vi "pp_sessList_save.vi"(8 "error in (no error)":errorcluster, 11 "Session List (Cannot Edit)":i32[](array[numeric])) -> (0 "error out":errorcluster, 3 "Session List File Path":path)   [LabVIEW 2013]
uses:
  <vilib>/Utility/file.llb/Write To Spreadsheet File (I64).vi
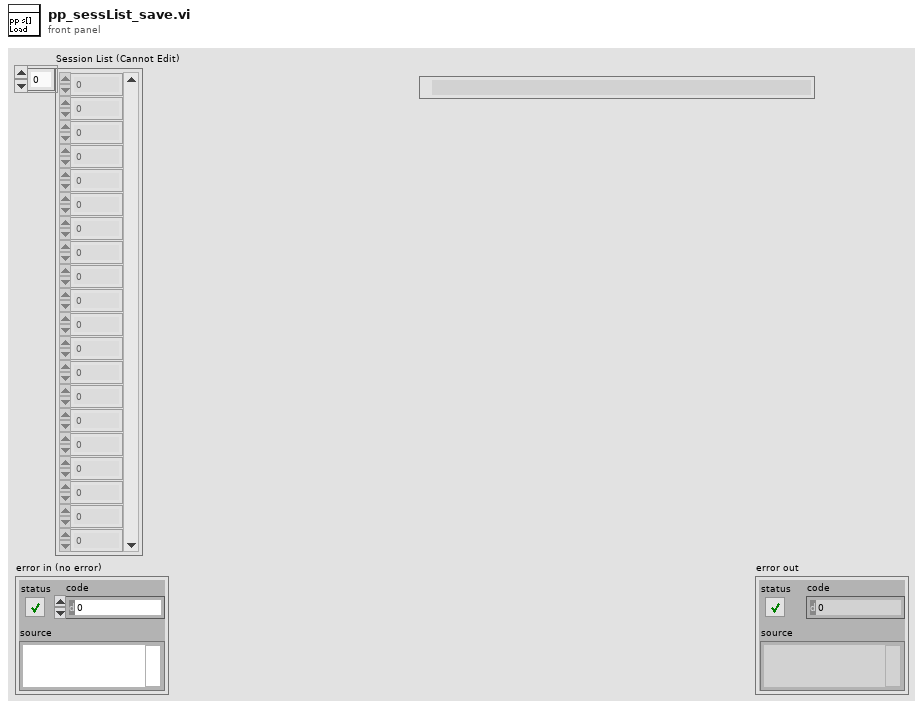
[diagram p1: front panel]
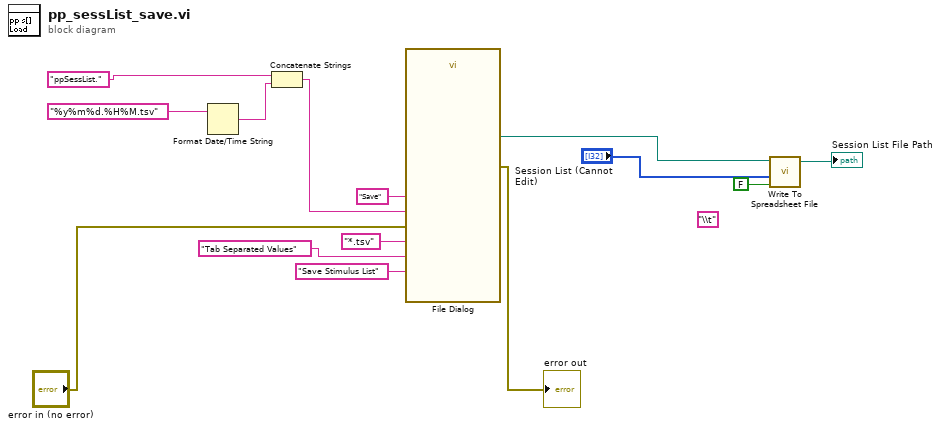
[diagram p0: block diagram]
diagram:
  (unwired) "\\t" ("delimiter (\\t)")
  n1 = Format Date/Time String(time format string (%c)="%y%m%d.%H%M.tsv") -> (date/time string=w10:string)  [unwired: 2 in]
  n2 = Concatenate Strings("ppSessList.", w10) -> (w9:string)
  n3 = call "File Dialog"("prompt"="Save Stimulus List", "button label"="Save", "default name"=w9, "error in"="error in (no error)", "pattern (all files)"="*.tsv", "pattern label"="Tab Separated Values") -> ("selected path"=w4:path, "error out"=→"error out":errorcluster)  [unwired: 6 in, 2 out]
  n4 = call-poly <vilib>:"Write To Spreadsheet File.vi"("append to file? (new file:F)"=FALSE, "1D data"="Session List (Cannot Edit)", "file path (dialog if empty)"=w4) -> ("new file path (Not A Path if cancelled)"=→"Session List File Path":path)  [unwired: 5 in]
